vi "Read Stop When Parent Stopped.vi"(11 "Actor in":refnum<class "Actor.lvclass">) -> (2 "Stop When Parent Stopped":bool)   [LabVIEW 2025, in "jettl.lvlib" / "Actor.lvclass"]
uses:
  Actor.lvclass
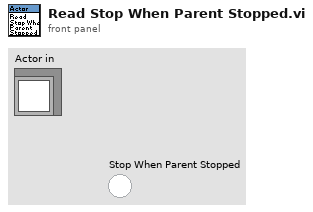
[diagram p1: front panel]
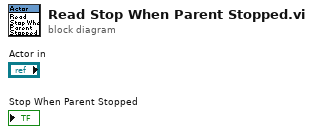
[diagram p0: block diagram]
diagram:
